vi "stage_control_mit_speichern.vi"() -> ()   [LabVIEW 2009]
uses:
  global_stage_initialised.vi
  <vilib>/Utility/inputDevices.llb/joystickAcquire.vi
  <vilib>/Utility/inputDevices.llb/closeJoystick.vi
panel:
  in  "Löschen":bool
  in  "Zeile":dbl
  out "Favoriten":i32[](listbox)
  in  "Laden":bool
  in  "Beschreibung":string
  in  "Speichern":bool
  in  "Wellenlänge":string
  in  "Joystick Index":i32
  in  "SN von Controller 1":string="0135500571"
  in  "Position auslesen":bool
  out "Joystickauslese":T1(ring)
  out "X-Achse pos/neg fahren":i32 min=-3000 max=2000
  out "Y-Achse pos/neg fahren":i32 min=-3000 max=2000
  in  "Schrittweite verringern":bool
  in  "Schrittweite erhoehen":bool
  out "Z-Achse pos fahren":bool
  out "Z-Achse neg fahren":bool
  out "Joystick ID":refnum<k1> caption="Geräte-ID"
  out "z-Achse":i32
  out "y-Achse":i32
  out "x-Achse":i32
  in  "Schrittweite [µm]":u16(ring) items=["500,0", "200,0", "100,0", "50,0", "20,0", "10,0", "5,0", "2,0", "1,0", "0,5", "0,1"]
  out "Aktuelle xyz-Position [mm]":dbl[](array[numeric]) format="%.5g"
  in  "Geschwindigkeit einstellen":bool
  in  "Ziel Geschwindigkeit [mm/s]":dbl=0.3 min=0.01 max=0.6 step=0.001 format="%.3g"
  out "Geschwindigkeit [mm/s]":dbl format="%.3g"
  in  "Negativer Schritt":bool[](array[boolean])
  in  "Positiver Schritt":bool[](array[boolean])
  out "error out":errorcluster
  out "Achse in \nBewegung":bool
  in  "Ziel xyz-Position [mm]":dbl[](array[numeric]) step=1e-05 format="%.5g"
  out "xyz-Bezeichnung":string[](array[string])=["x [mm]", "y [mm]", "z [mm]"]
  in  "Bühnen schließen":bool
  out "Bühnen\ninitialisiert":bool
  # "Steuerung der 3D-Translationsbühne von PI"
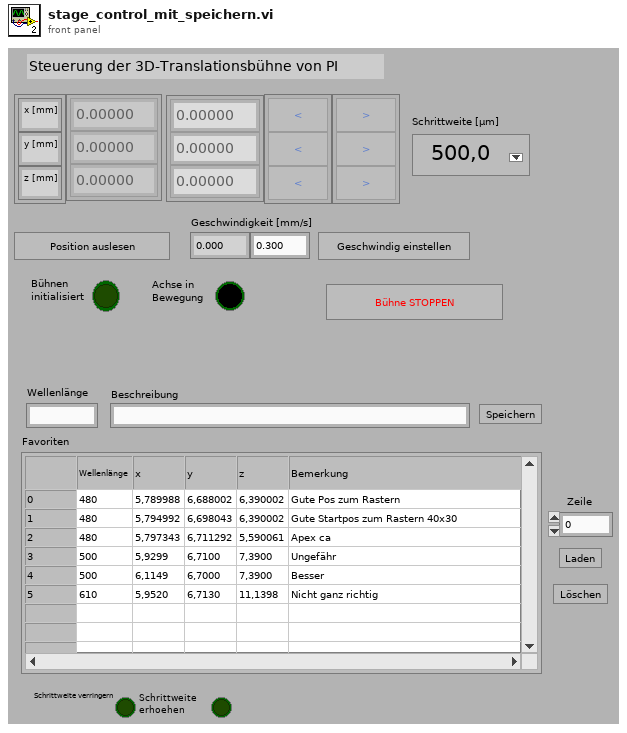
[diagram p1: front panel]
types:
  T1 = enum16{"Nichts tun", "X-Achse", "Y-Achse", "Z-Achse positiv", "Z-Achse negativ", "Schrittweite erhoehen", "Schrittweite verringern"}
  T2 = cluster{"Objektnamen":string[][], "Zeilentitel":string[], "Spaltentitel":string[]}
  T3 = cluster{"X axis":i32, "Y axis":i32, "Z axis":i32, "X axis rotation":i32, "Y axis rotation":i32, "Z axis rotation":i32, "U axis":i32, "V axis":i32}
  T4 = cluster{"button 1":bool, "button 2":bool, "button 3":bool, "button 4":bool, "button 5":bool, "button 6":bool, "button 7":bool, "button 8":bool, "button 9":bool, "button 10":bool, "button 11":bool, "button 12":bool, "button 13":bool, "button 14":bool, "button 15":bool, "button 16":bool, "button 17":bool, "button 18":bool, "button 19":bool, "button 20":bool, "button 21":bool, "button 22":bool, "button 23":bool, "button 24":bool, "button 25":bool, "button 26":bool, "button 27":bool, "button 28":bool, "button 29":bool, "button 30":bool, "button 31":bool, "button 32":bool}
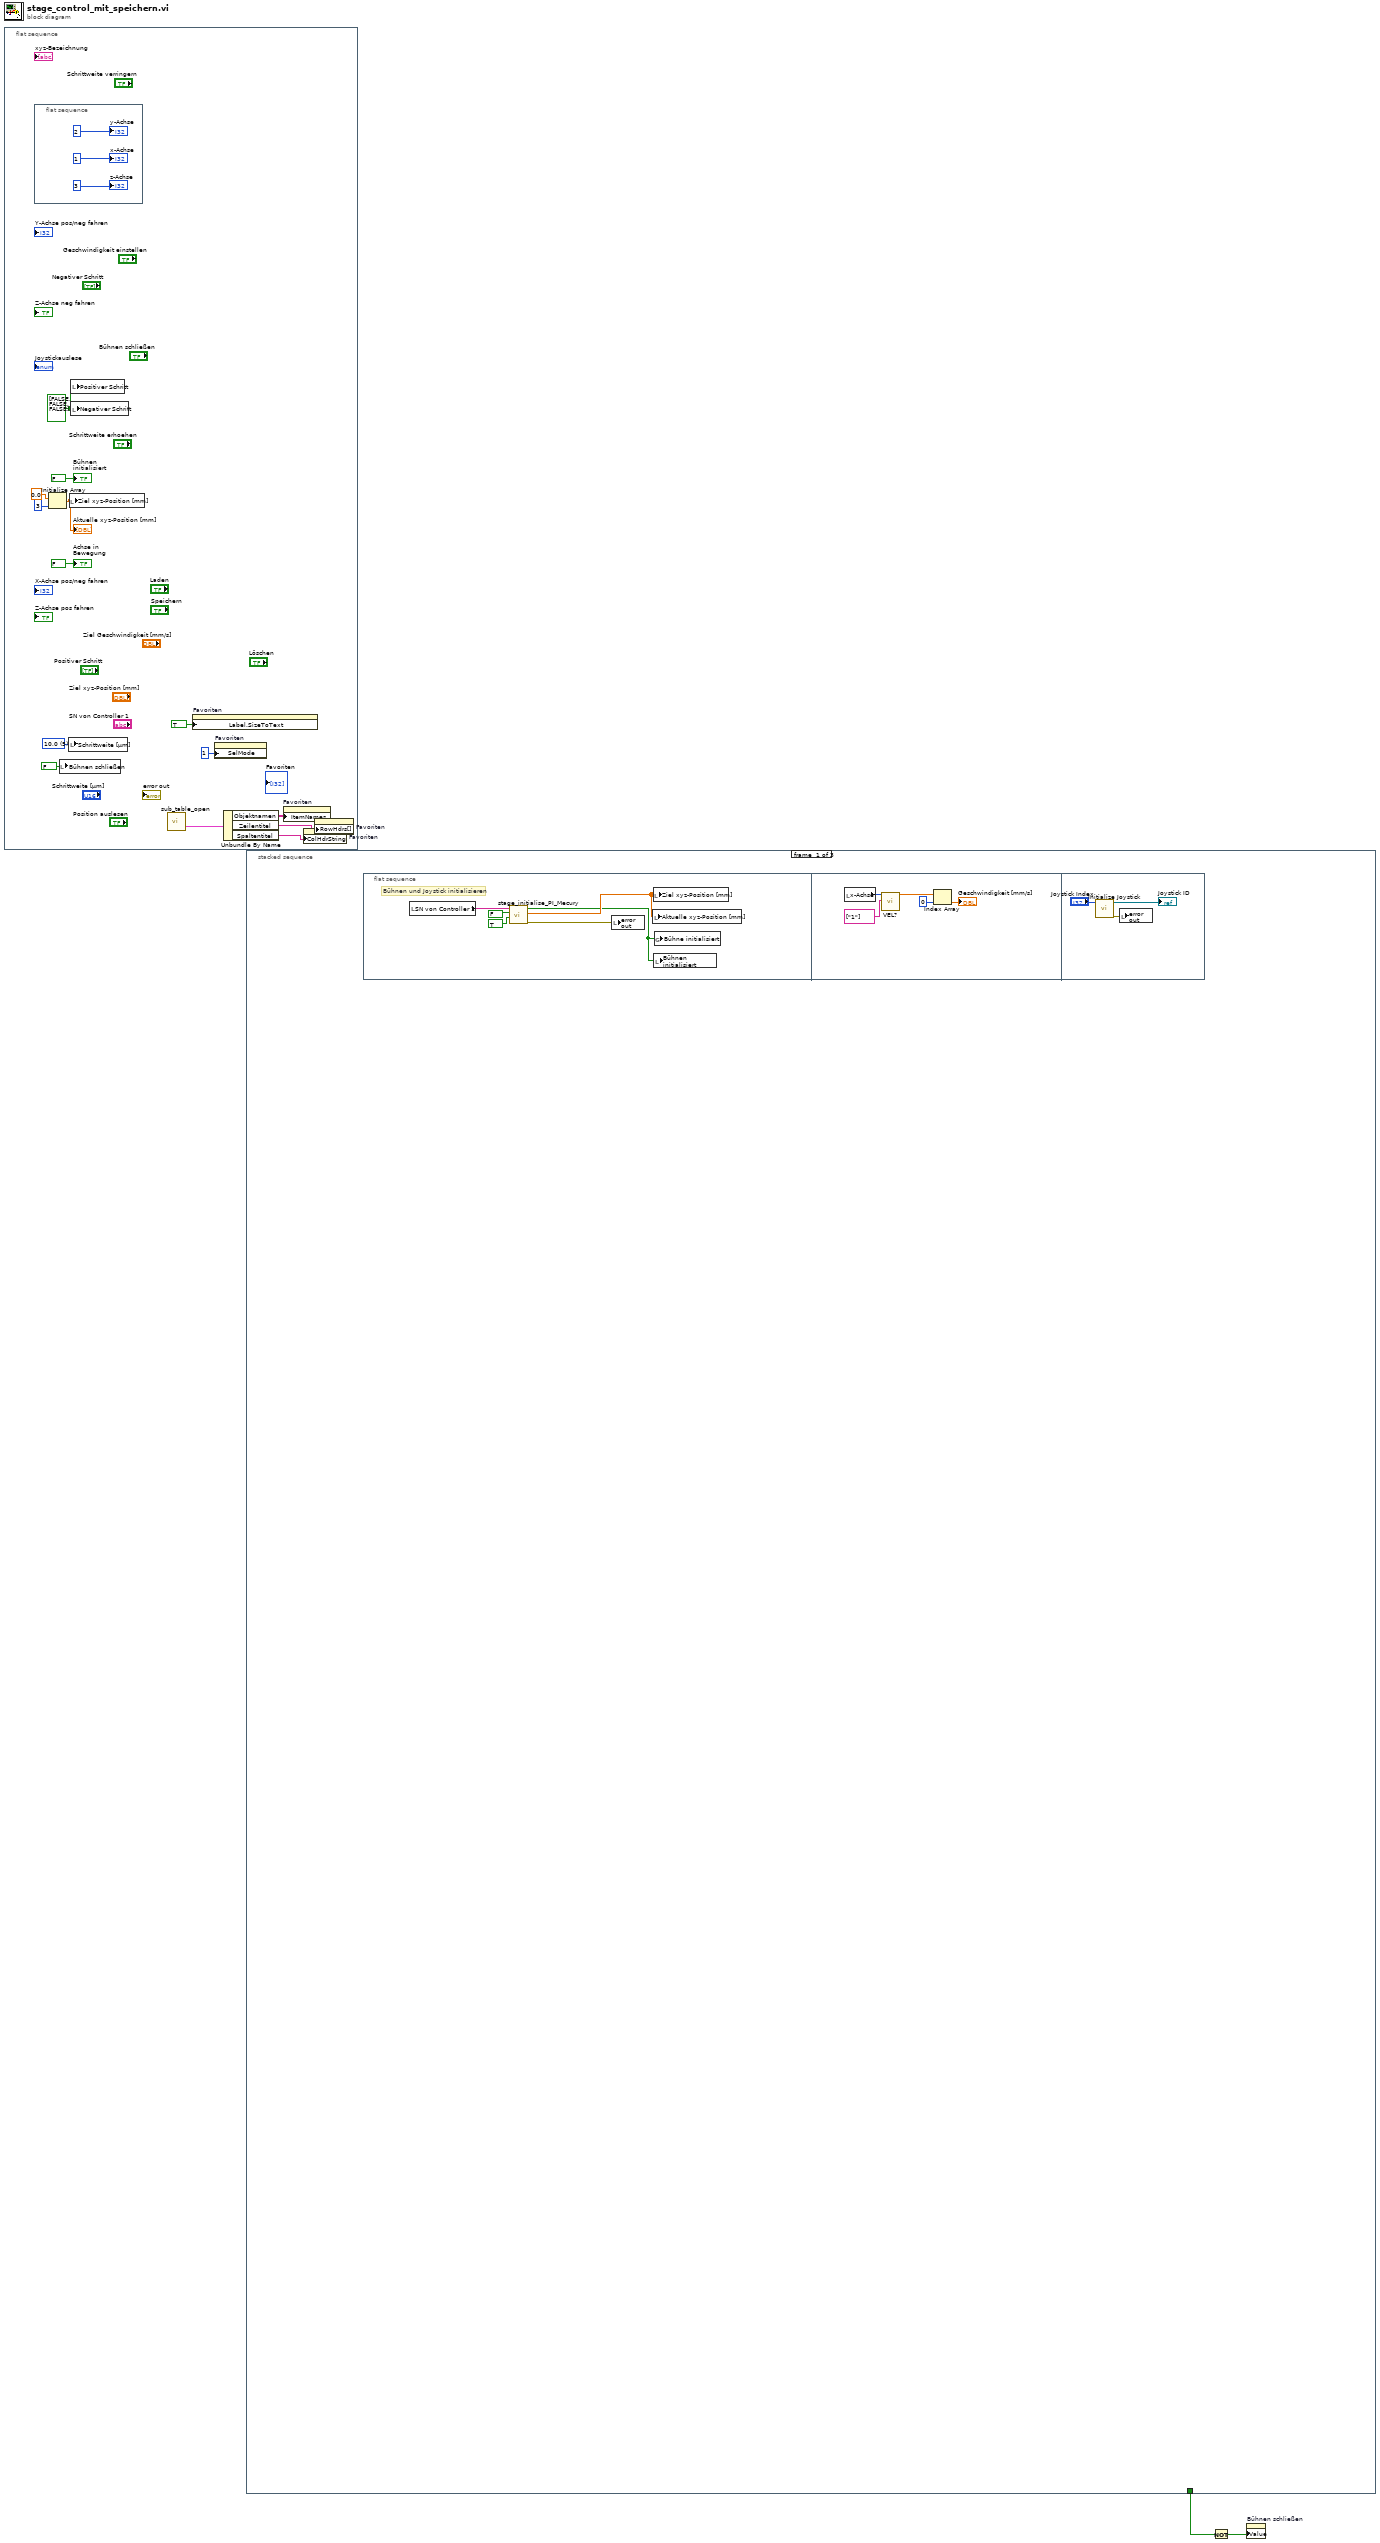
[diagram p0: block diagram]
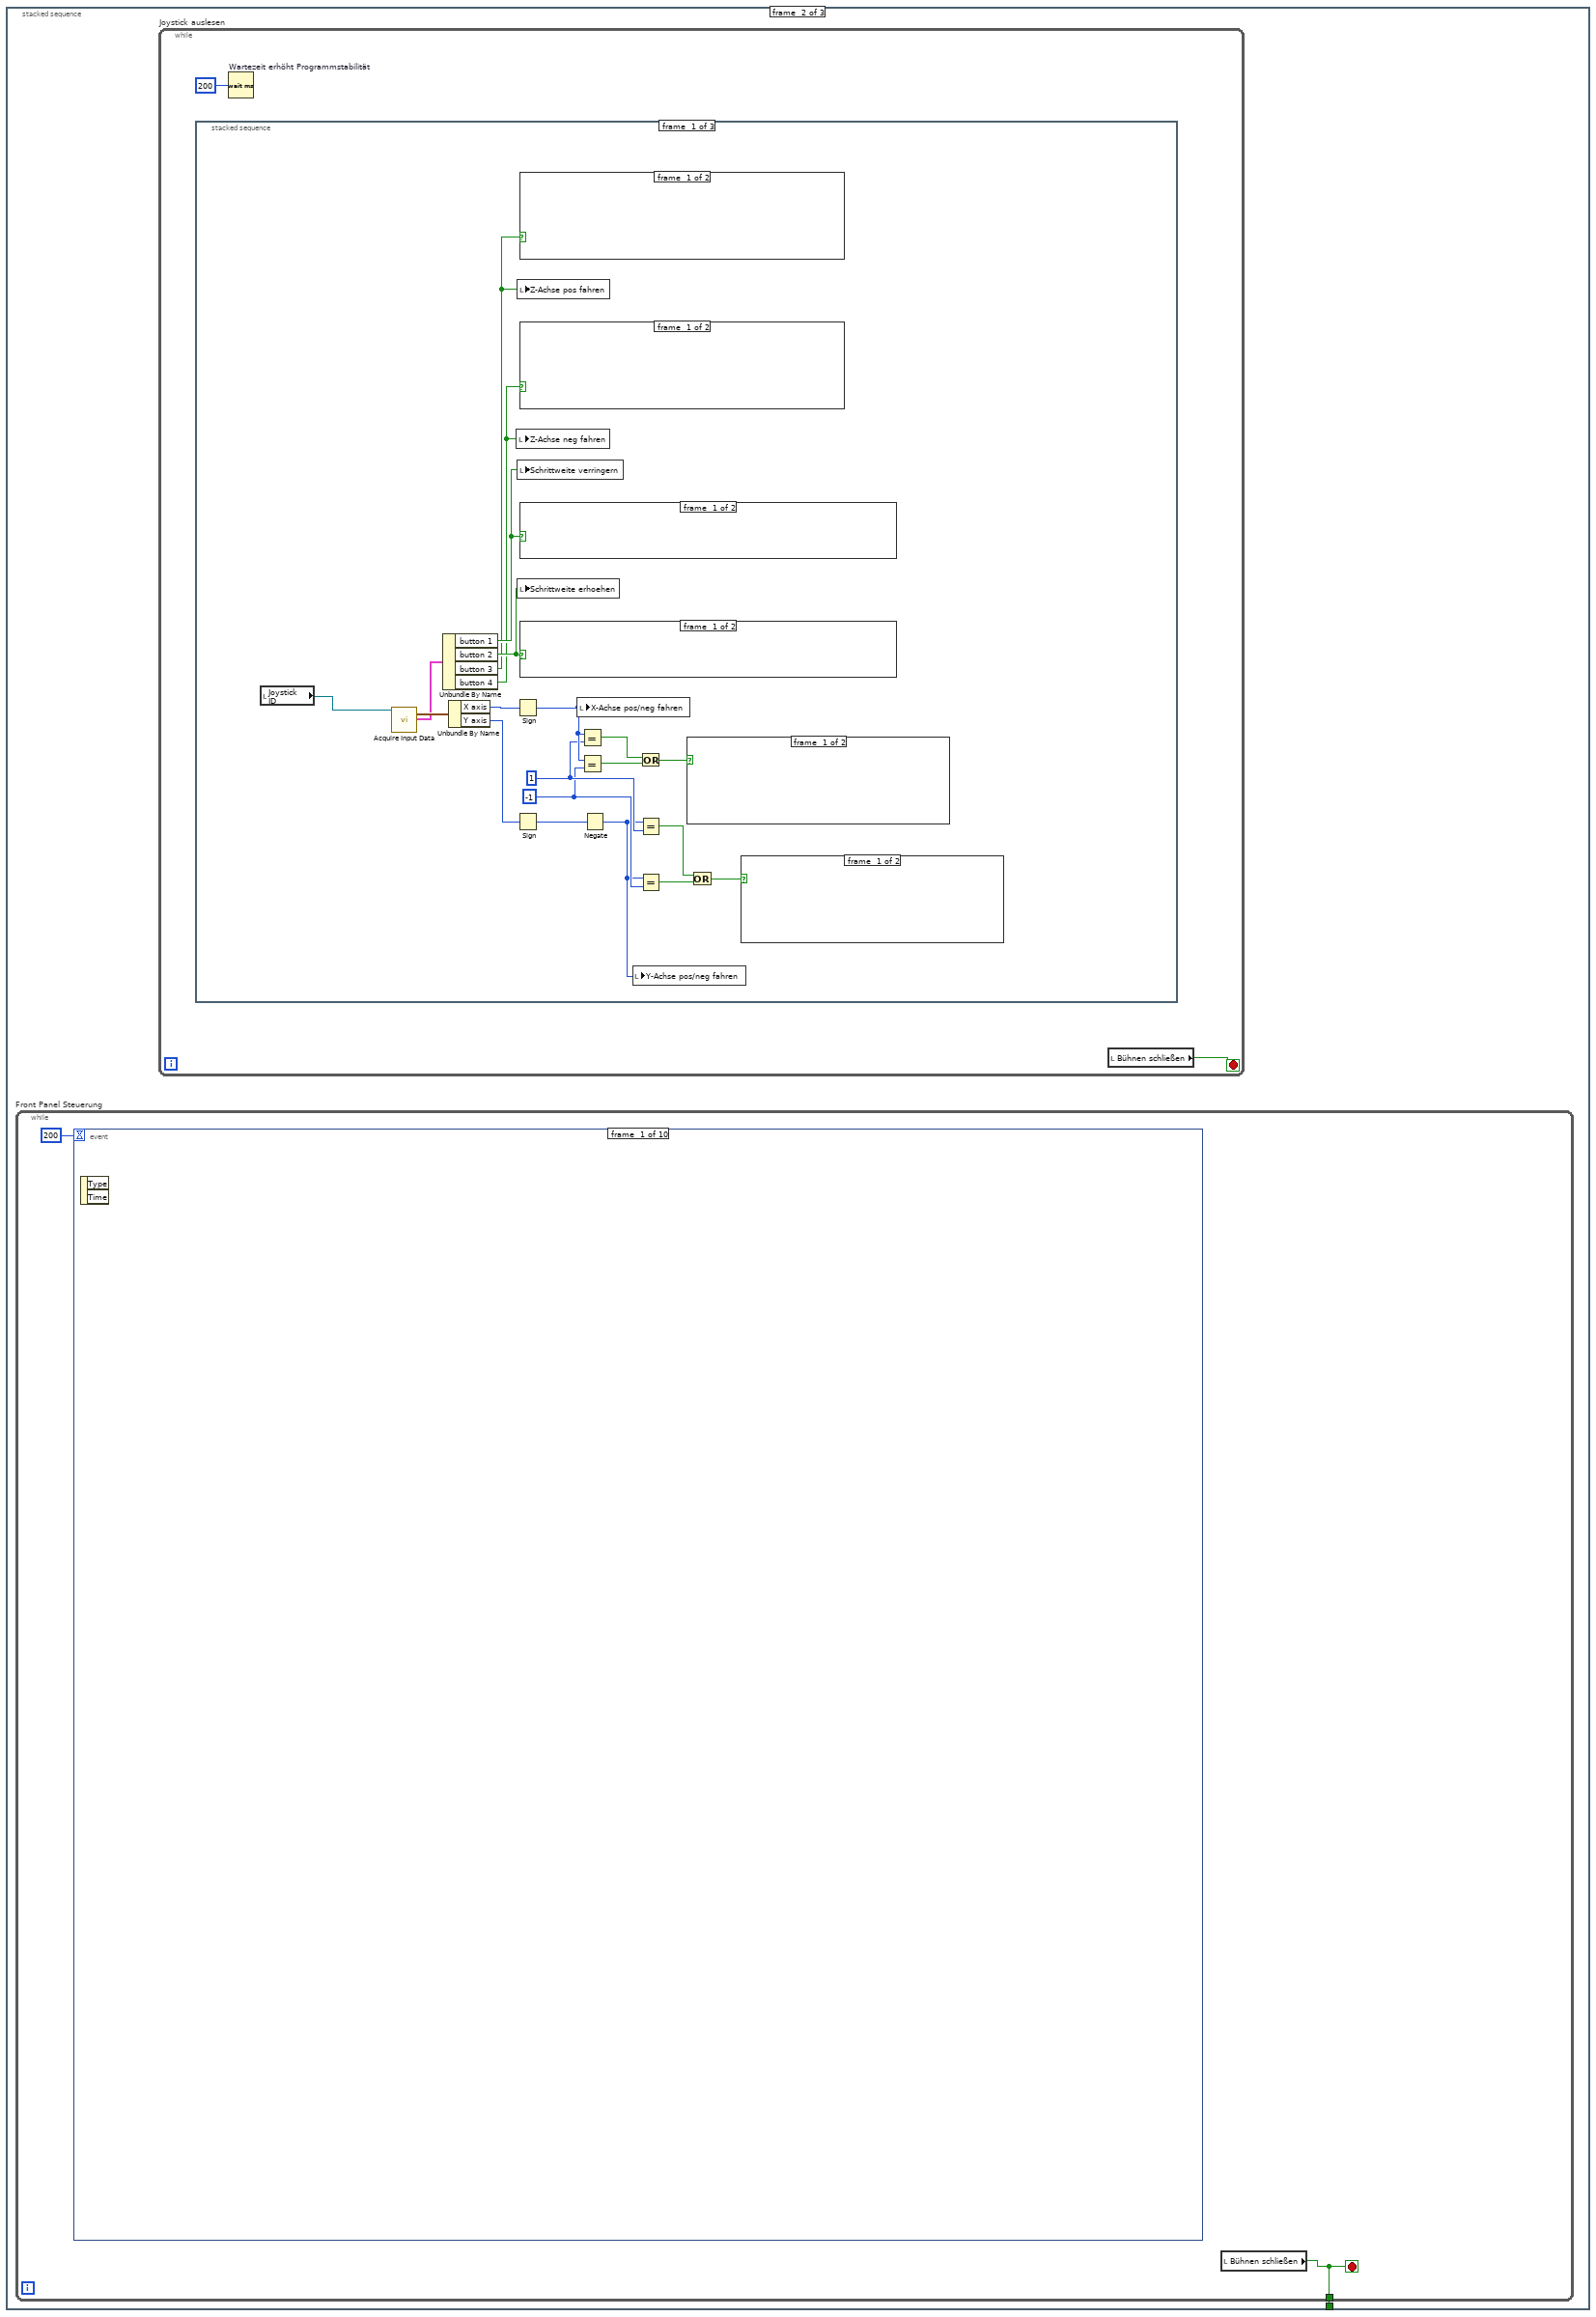
[diagram p2: hidden frame]
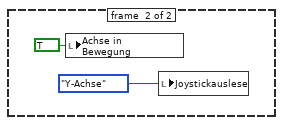
[diagram p3: hidden frame]
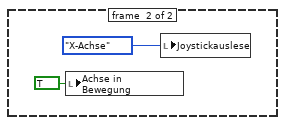
[diagram p4: hidden frame]
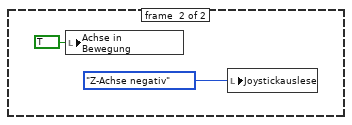
[diagram p5: hidden frame]
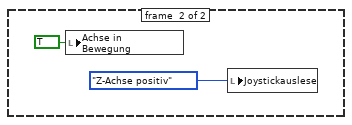
[diagram p6: hidden frame]
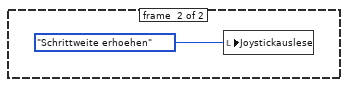
[diagram p7: hidden frame]
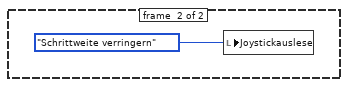
[diagram p8: hidden frame]
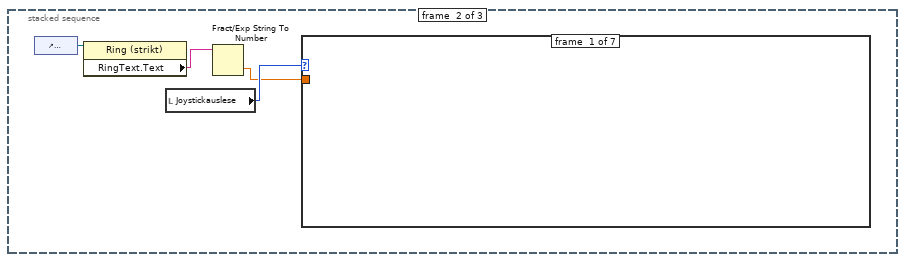
[diagram p9: hidden frame]
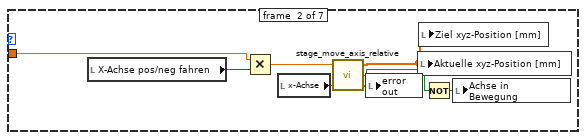
[diagram p10: hidden frame]
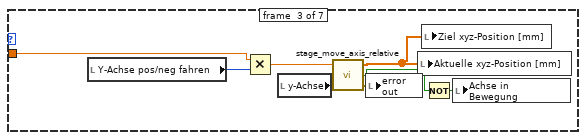
[diagram p11: hidden frame]
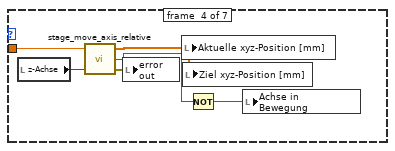
[diagram p12: hidden frame]
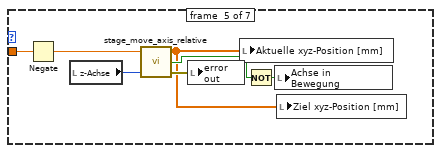
[diagram p13: hidden frame]
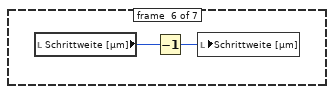
[diagram p14: hidden frame]
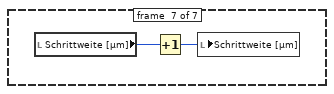
[diagram p15: hidden frame]
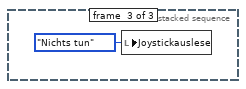
[diagram p16: hidden frame]
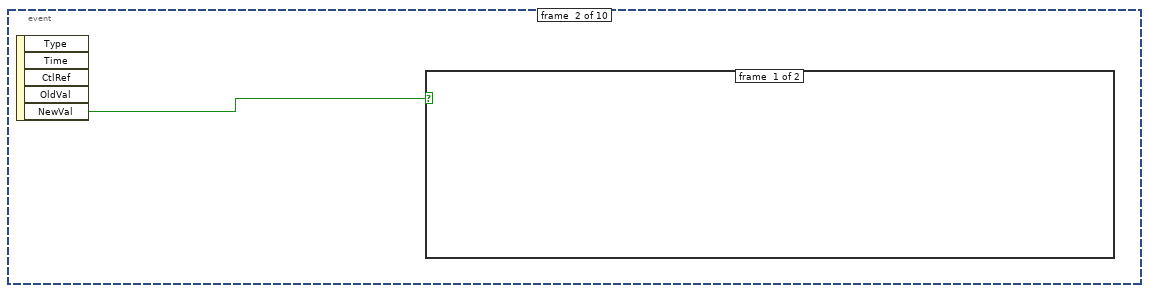
[diagram p17: hidden frame]
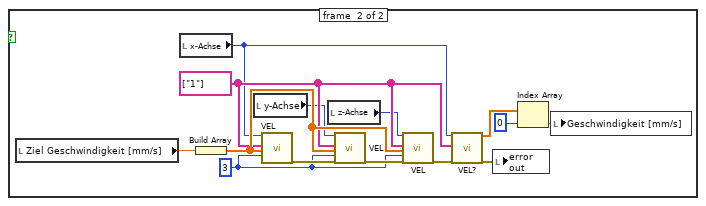
[diagram p18: hidden frame]
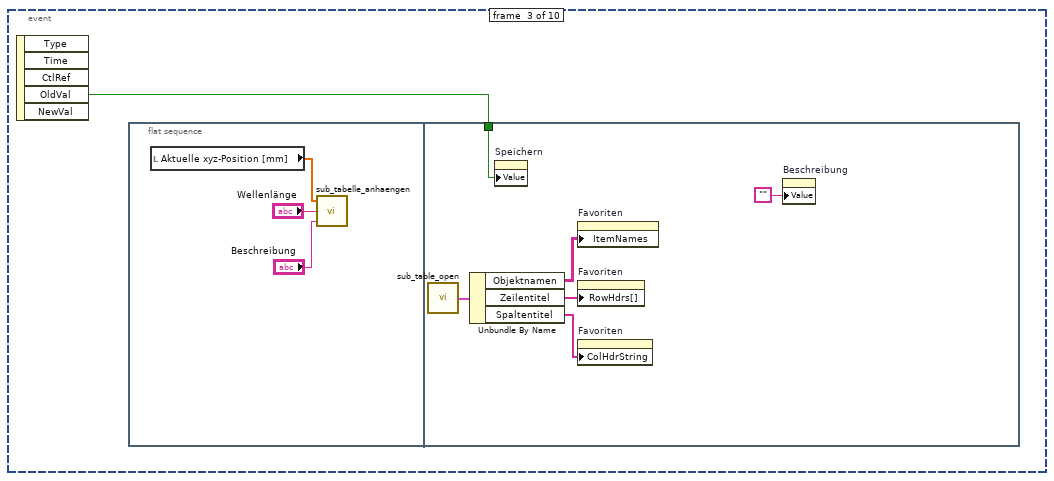
[diagram p19: hidden frame]
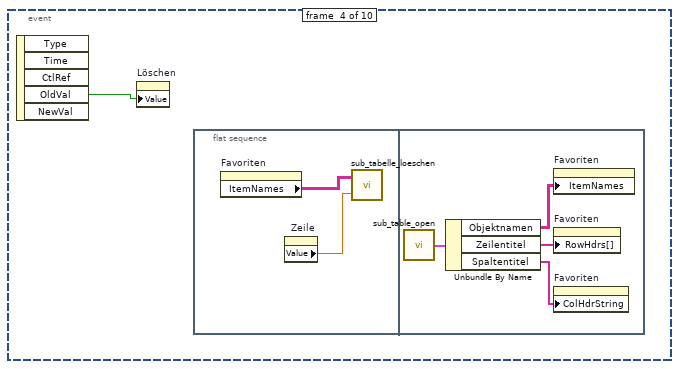
[diagram p20: hidden frame]
diagram:
  n1 = flat-sequence {
    frame #0 {
      w15 = u16 5 items=["500,0", "200,0", "100,0", "50,0", "20,0", "10,0", "5,0", "2,0", "1,0", "0,5"] ("Schrittweite [µm]")
      w11 = bool[] [FALSE, FALSE, FALSE] ("Positiver Schritt")
      n2 = flat-sequence {
        frame #0 {
          "x-Achse" <- 1 ("x-Achse")
          "y-Achse" <- 2 ("y-Achse")
          "z-Achse" <- 3 ("z-Achse")
        }
      }
      n3 = Initialize Array(0.0 ("Element"), 3 ("Dimension")) -> (w14:dbl[])
      "Aktuelle xyz-Position [mm]" <- w14
      n4 = local write "Bühnen schließen"(FALSE ("Bühnen schließen")) -> ()
      n5 = local write "Schrittweite [µm]"(w15) -> ()
      n6 = local write "Ziel xyz-Position [mm]"(w14) -> ()
      n7 = local write "Positiver Schritt"(w11) -> ()
      n8 = local write "Negativer Schritt"(w11) -> ()
      n9 = call "sub_table_open.vi"() -> ("Cluster (Ausgang)"=w6:T2)  [unwired: 1 in]
      n10 = property on="Favoriten" class="MehrSpaltListenfeld (strikt)"("Label.SizeToText"=TRUE ("Beschriftung.Größe an Text anpassen?")) -> ()  [unwired: 2 in, 2 out]
      n11 = property on="Favoriten" class="MehrSpaltListenfeld (strikt)"("SelMode"=1 ("Auswahlmodus")) -> ()  [unwired: 2 in, 2 out]
      n12 = Unbundle By Name(w6) -> ("Objektnamen"=w5:string[][], "Zeilentitel"=w3:string[], "Spaltentitel"=w4:string[])
      n13 = property on="Favoriten" class="MehrSpaltListenfeld (strikt)"("ItemNames"=w5) -> ()  [unwired: 2 in, 2 out]
      n14 = property on="Favoriten" class="MehrSpaltListenfeld (strikt)"("ColHdrString"=w4) -> ()  [unwired: 2 in, 2 out]
      n15 = property on="Favoriten" class="MehrSpaltListenfeld (strikt)"("RowHdrs[]"=w3) -> ()  [unwired: 2 in, 2 out]
      "Bühnen\ninitialisiert" <- FALSE ("Bühnen initialisiert")
      "Achse in \nBewegung" <- FALSE ("x-Achse in Bewegung")
    }
  }
  n16 = stacked-sequence {
    tunnel: [_ w34 _] -> w2
    frame #0 {
      n17 = flat-sequence {
        frame #0 {
          # "Bühnen und Joystick initialisieren"
          n18 = local read "SN von Controller 1"() -> (w20:string)
          n19 = call "stage_initialise_PI_Mecury.vi"("Referenz Modus"=TRUE, "Referenzierung erzwingen"=FALSE, "SN von Controller 1"=w20) -> ("error out"=w23:errorcluster, "Aktuelle xyz-Position"=w22:dbl[], "Bühnen initialisiert"=w21:bool)  [unwired: 6 in]
          n20 = local write "error out"(w23) -> ()
          n21 = local write "Aktuelle xyz-Position [mm]"(w22) -> ()
          n22 = local write "Ziel xyz-Position [mm]"(w22) -> ()
          n23 = local write "Bühnen\ninitialisiert"(w21) -> ()
          n24 = global write "global_stage_initialised.vi" "Bühne initialisiert"(w21) -> ()
        }
        frame #1 {
          n25 = local read "x-Achse"() -> (w26:i32)
          n26 = call "VEL?.vi"("System no."=w26, "Axes to query"=string[] ["1"]) -> ("Velocity"=w27:dbl[])  [unwired: 16 in, 1 out]
          n27 = Index Array(array=w27, index=0 ("Index")) -> (element=→"Geschwindigkeit [mm/s]":dbl)
        }
        frame #2 {
          n28 = call <vilib>:"Initialize Joystick.vi"("device index"="Joystick Index") -> ("error out"=w32:errorcluster, "device ID"=→"Joystick ID":refnum<k1>)  [unwired: 9 in]
          n29 = local write "error out"(w32) -> ()
        }
      }
    }
    frame #1 {
      n30 = while "Front Panel Steuerung" {
        tunnel: [w105] -> w34
        stop <- w105 stop-if-true
        n31 = event shown="[2] \"Speichern\": Wertänderung" {
          selector: _ -> [_ _ _ _ _ _ _ _ _ _]
          dyn-events: _ -> [_ _ _ _ _ _ _ _ _ _]
          timeout: 200 -> [_ _ _ _ _ _ _ _ _ _]
          event #0 {
            n32 = event-data() -> ()  [unwired: 1 in, 2 out]
          }
          event #1 {
            n33 = event-data() -> ("NewVal"=w107:bool)  [unwired: 1 in, 4 out]
            n34 = case shown="True" w107 {
              frame #0 {
              }
              frame #1 {
                w118 = i16 3 ("No.of digits")
                w114 = string[] ["1"] ("Axes to set")
                n35 = local read "Ziel Geschwindigkeit [mm/s]"() -> (w119:dbl)
                n36 = local read "x-Achse"() -> (w110:i32)
                n37 = Build Array(w119) -> (w117:dbl[])
                n38 = local read "y-Achse"() -> (w109:i32)
                n39 = call "VEL.vi"("System no."=w110, "Axes to set"=w114, "Velocity values"=w117, "No.of digits"=w118) -> ("error out"=w121:errorcluster)  [unwired: 14 in, 1 out]
                n40 = local read "z-Achse"() -> (w108:i32)
                n41 = call "VEL.vi"("System no."=w109, "Axes to set"=w114, "Velocity values"=w117, "No.of digits"=w118, "error in"=w121) -> ("error out"=w120:errorcluster)  [unwired: 13 in, 1 out]
                n42 = call "VEL.vi"("System no."=w108, "Axes to set"=w114, "Velocity values"=w117, "No.of digits"=w118, "error in"=w120) -> ("error out"=w115:errorcluster)  [unwired: 13 in, 1 out]
                n43 = call "VEL?.vi"("System no."=w110, "Axes to query"=w114, "error in"=w115) -> ("Velocity"=w112:dbl[], "error out"=w116:errorcluster)  [unwired: 15 in]
                n44 = local write "error out"(w116) -> ()
                n45 = Index Array(array=w112, index=0 ("Index")) -> (element=w113:dbl)
                n46 = local write "Geschwindigkeit [mm/s]"(w113) -> ()
              }
            }
          }
          event #2 {
            n47 = event-data() -> ("OldVal"=w122:bool)  [unwired: 1 in, 4 out]
            n48 = flat-sequence {
              tunnel: w122 -> [w130]
              frame #0 {
                n49 = local read "Aktuelle xyz-Position [mm]"() -> (w123:dbl[])
                n50 = call "sub_tabelle_anhaengen.vi"("Beschreibung"="Beschreibung", "Wellenlänge"="Wellenlänge", "Aktuelle xyz-Position [mm]"=w123) -> ()
              }
              frame #1 {
                n51 = call "sub_table_open.vi"() -> ("Cluster (Ausgang)"=w129:T2)  [unwired: 1 in]
                n52 = Unbundle By Name(w129) -> ("Objektnamen"=w128:string[][], "Zeilentitel"=w127:string[], "Spaltentitel"=w126:string[])
                n53 = property on="Speichern" class="Boolesch (strikt)"("Value"=w130) -> ()  [unwired: 2 in, 2 out]
                n54 = property on="Favoriten" class="MehrSpaltListenfeld (strikt)"("ItemNames"=w128) -> ()  [unwired: 2 in, 2 out]
                n55 = property on="Favoriten" class="MehrSpaltListenfeld (strikt)"("RowHdrs[]"=w127) -> ()  [unwired: 2 in, 2 out]
                n56 = property on="Favoriten" class="MehrSpaltListenfeld (strikt)"("ColHdrString"=w126) -> ()  [unwired: 2 in, 2 out]
                n57 = property on="Beschreibung" class="Str"("Value"="") -> ()  [unwired: 2 in, 2 out]
              }
            }
          }
          event #3 {
            n58 = event-data() -> ("OldVal"=w132:bool)  [unwired: 1 in, 4 out]
            n59 = property on="Löschen" class="Boolesch (strikt)"("Value"=w132) -> ()  [unwired: 2 in, 2 out]
            n60 = flat-sequence {
              frame #0 {
                n61 = property on="Favoriten" class="MehrSpaltListenfeld (strikt)"() -> ("ItemNames"=w133:string[][])  [unwired: 2 in, 2 out]
                n62 = property on="Zeile" class="DigitalWert (strikt)"() -> ("Value"=w134:dbl)  [unwired: 2 in, 2 out]
                n63 = call "sub_tabelle_loeschen.vi"("Numerisches Element"=w134, "Array"=w133) -> ()  [unwired: 1 in]
              }
              frame #1 {
                n64 = call "sub_table_open.vi"() -> ("Cluster (Ausgang)"=w138:T2)  [unwired: 1 in]
                n65 = Unbundle By Name(w138) -> ("Objektnamen"=w135:string[][], "Zeilentitel"=w137:string[], "Spaltentitel"=w136:string[])
                n66 = property on="Favoriten" class="MehrSpaltListenfeld (strikt)"("ItemNames"=w135) -> ()  [unwired: 2 in, 2 out]
                n67 = property on="Favoriten" class="MehrSpaltListenfeld (strikt)"("RowHdrs[]"=w137) -> ()  [unwired: 2 in, 2 out]
                n68 = property on="Favoriten" class="MehrSpaltListenfeld (strikt)"("ColHdrString"=w136) -> ()  [unwired: 2 in, 2 out]
              }
            }
          }
          event #4 {
            n69 = event-data() -> ("OldVal"=w141:bool)  [unwired: 1 in, 4 out]
            n70 = local write "Laden"(w141) -> ()
            n71 = property on="Favoriten" class="MehrSpaltListenfeld (strikt)"() -> ("ItemNames"=w140:string[][])  [unwired: 2 in, 2 out]
            n72 = call "sub_table_laden.vi"("Zeile"="Zeile", "ItemNames"=w140) -> ("Array"=w139:dbl[])
            n73 = property on="Ziel xyz-Position [mm]" class="Arr (strikt)"("Val(Sgnl)"=w139) -> ()  [unwired: 2 in, 2 out]
          }
          event #5 {
            n74 = event-data() -> ("NewVal"=w143:bool)  [unwired: 1 in, 4 out]
            n75 = case shown="True" w143 {
              frame #0 {
              }
              frame #1 {
                n76 = call "stage_get_current_xyz.vi"() -> ("error out"=w145:errorcluster, "Aktuelle xyz-Position OUT [mm]"=w144:dbl[])  [unwired: 3 in]
                n77 = local write "Aktuelle xyz-Position [mm]"(w144) -> ()
                n78 = local write "error out"(w145) -> ()
                n79 = local write "Ziel xyz-Position [mm]"(w144) -> ()
              }
            }
          }
          event #6 {
            n80 = event-data() -> ("OldVal"=w147:dbl[], "NewVal"=w146:dbl[])  [unwired: 1 in, 3 out]
            n81 = flat-sequence {
              tunnel: [w153] -> w150
              tunnel: [w152] -> w149
              tunnel: [w151] -> w148
              tunnel: w147 -> [w155]
              tunnel: w146 -> [w154]
              tunnel: w150 -> [w169]
              tunnel: w149 -> [w168]
              tunnel: w148 -> [w167]
              frame #0 {
                w158 = 2 ("Index")
                w157 = 1 ("Index")
                w156 = 0 ("Index")
                # "Änderung des Ziels: Entscheide welche Achse gefahren werden soll"
                n82 = local write "Achse in \nBewegung"(TRUE ("x-Achse in Bewegung")) -> ()
                n83 = Index Array(array=w155, index #1=w156, index #2=w157, index #3=w158) -> (element #1=w159:dbl, element #2=w160:dbl, element #3=w163:dbl)
                n84 = Index Array(array=w154, index #1=w156, index #2=w157, index #3=w158) -> (element #1=w164:dbl, element #2=w161:dbl, element #3=w162:dbl)
                n85 = Not Equal?(x=w159, y=w164) -> (x != y?=w153:bool)
                n86 = Not Equal?(x=w160, y=w161) -> (x != y?=w152:bool)
                n87 = Not Equal?(x=w163, y=w162) -> (x != y?=w151:bool)
              }
              frame #1 {
                n88 = local read "Ziel xyz-Position [mm]"() -> (w166:dbl[])
                n89 = case shown="True" w169 {
                  tunnel: w166 -> [_ w186]
                  frame #0 {
                  }
                  frame #1 {
                    n90 = local read "x-Achse"() -> (w184:i32)
                    n91 = call "stage_move_axis_absolute.vi"("Ziel xyz IN [mm]"=w186, "Achse"=w184) -> ("error out"=w187:errorcluster, "Fertig?"=w185:bool, "Ziel xyz OUT [mm]"=w182:dbl[])  [unwired: 1 in]
                    n92 = local write "Aktuelle xyz-Position [mm]"(w182) -> ()
                    n93 = local write "Ziel xyz-Position [mm]"(w182) -> ()
                    n94 = local write "error out"(w187) -> ()
                    n95 = Not(x=w185) -> (.not. x?=w183:bool)
                    n96 = local write "Achse in \nBewegung"(w183) -> ()
                  }
                }
                n97 = case shown="True" w168 {
                  tunnel: w166 -> [_ w180]
                  frame #0 {
                  }
                  frame #1 {
                    n98 = local read "y-Achse"() -> (w178:i32)
                    n99 = call "stage_move_axis_absolute.vi"("Ziel xyz IN [mm]"=w180, "Achse"=w178) -> ("error out"=w181:errorcluster, "Fertig?"=w179:bool, "Ziel xyz OUT [mm]"=w176:dbl[])  [unwired: 1 in]
                    n100 = local write "Aktuelle xyz-Position [mm]"(w176) -> ()
                    n101 = local write "Ziel xyz-Position [mm]"(w176) -> ()
                    n102 = local write "error out"(w181) -> ()
                    n103 = Not(x=w179) -> (.not. x?=w177:bool)
                    n104 = local write "Achse in \nBewegung"(w177) -> ()
                  }
                }
                n105 = case shown="True" w167 {
                  tunnel: w166 -> [_ w173]
                  frame #0 {
                  }
                  frame #1 {
                    n106 = local read "z-Achse"() -> (w172:i32)
                    n107 = call "stage_move_axis_absolute.vi"("Ziel xyz IN [mm]"=w173, "Achse"=w172) -> ("error out"=w175:errorcluster, "Fertig?"=w174:bool, "Ziel xyz OUT [mm]"=w170:dbl[])  [unwired: 1 in]
                    n108 = local write "Aktuelle xyz-Position [mm]"(w170) -> ()
                    n109 = local write "Ziel xyz-Position [mm]"(w170) -> ()
                    n110 = local write "error out"(w175) -> ()
                    n111 = Not(x=w174) -> (.not. x?=w171:bool)
                    n112 = local write "Achse in \nBewegung"(w171) -> ()
                  }
                }
              }
            }
          }
          event #7 {
            n113 = event-data() -> ("Row"=w188:i32)  [unwired: 1 in, 7 out]
            n114 = local write "Zeile"(w188) -> ()
          }
          event #8 {
            n115 = event-data() -> ("NewVal"=w193:bool[])  [unwired: 1 in, 4 out]
            n116 = Index Array(array=w193, index #1=0 ("Index"), index #2=1 ("Index"), index #3=2 ("Index")) -> (element #1=w191:bool, element #2=w190:bool, element #3=w189:bool)
            n117 = Compound Arithmetic op=OR(w191, w190, w189) -> (w192:bool)
            n118 = case shown="True" w192 {
              tunnel: w191 -> [_ w199]
              tunnel: w190 -> [_ w198]
              tunnel: w189 -> [_ w197]
              frame #0 {
              }
              frame #1 {
                n119 = flat-sequence {
                  tunnel: [w202] -> w200
                  tunnel: w200 -> [w208]
                  tunnel: w199 -> [w207]
                  tunnel: w198 -> [w206]
                  tunnel: w197 -> [w205]
                  frame #0 {
                    n120 = local write "Achse in \nBewegung"(TRUE ("Achse in Bewegung")) -> ()
                    n121 = control-ref of="Schrittweite [µm]"() -> (w204:refnum<vi>)
                    n122 = property class="Ring (strikt)"(reference=w204) -> ("RingText.Text"=w203:string)  [unwired: 1 in, 2 out]
                    n123 = Fract/Exp String To Number(string=w203) -> (number=w202:dbl)  [unwired: 3 in, 1 out]
                  }
                  frame #1 {
                    n124 = local read "x-Achse"() -> (w211:i32)
                    n125 = local read "y-Achse"() -> (w209:i32)
                    n126 = local read "z-Achse"() -> (w210:i32)
                    n127 = case shown="True" w205 {
                      tunnel: w210 -> [_ w217]
                      tunnel: w208 -> [_ w213]
                      frame #0 {
                      }
                      frame #1 {
                        n128 = call "stage_move_axis_relative.vi"("Achse"=w217, "Schrittweite [µm]"=w213) -> ("error out"=w216:errorcluster, "Fertig?"=w215:bool, "xyz-Position OUT [mm]"=w212:dbl[])  [unwired: 1 in]
                        n129 = local write "Aktuelle xyz-Position [mm]"(w212) -> ()
                        n130 = local write "Ziel xyz-Position [mm]"(w212) -> ()
                        n131 = local write "error out"(w216) -> ()
                        n132 = Not(x=w215) -> (.not. x?=w214:bool)
                        n133 = local write "Achse in \nBewegung"(w214) -> ()
                      }
                    }
                    n134 = case shown="True" w206 {
                      tunnel: w209 -> [_ w222]
                      tunnel: w208 -> [_ w219]
                      frame #0 {
                      }
                      frame #1 {
                        n135 = call "stage_move_axis_relative.vi"("Achse"=w222, "Schrittweite [µm]"=w219) -> ("error out"=w223:errorcluster, "Fertig?"=w221:bool, "xyz-Position OUT [mm]"=w218:dbl[])  [unwired: 1 in]
                        n136 = local write "Aktuelle xyz-Position [mm]"(w218) -> ()
                        n137 = local write "Ziel xyz-Position [mm]"(w218) -> ()
                        n138 = local write "error out"(w223) -> ()
                        n139 = Not(x=w221) -> (.not. x?=w220:bool)
                        n140 = local write "Achse in \nBewegung"(w220) -> ()
                      }
                    }
                    n141 = case shown="True" w207 {
                      tunnel: w211 -> [_ w228]
                      tunnel: w208 -> [_ w225]
                      frame #0 {
                      }
                      frame #1 {
                        n142 = call "stage_move_axis_relative.vi"("Achse"=w228, "Schrittweite [µm]"=w225) -> ("error out"=w229:errorcluster, "Fertig?"=w227:bool, "xyz-Position OUT [mm]"=w224:dbl[])  [unwired: 1 in]
                        n143 = local write "Aktuelle xyz-Position [mm]"(w224) -> ()
                        n144 = local write "Ziel xyz-Position [mm]"(w224) -> ()
                        n145 = local write "error out"(w229) -> ()
                        n146 = Not(x=w227) -> (.not. x?=w226:bool)
                        n147 = local write "Achse in \nBewegung"(w226) -> ()
                      }
                    }
                  }
                }
              }
            }
          }
          event #9 {
            n148 = event-data() -> ("NewVal"=w234:bool[])  [unwired: 1 in, 4 out]
            n149 = Index Array(array=w234, index #1=0 ("Index"), index #2=1 ("Index"), index #3=2 ("Index")) -> (element #1=w232:bool, element #2=w231:bool, element #3=w230:bool)
            n150 = Compound Arithmetic op=OR(w232, w231, w230) -> (w233:bool)
            n151 = case shown="True" w233 {
              tunnel: w232 -> [_ w240]
              tunnel: w231 -> [_ w239]
              tunnel: w230 -> [_ w238]
              frame #0 {
              }
              frame #1 {
                n152 = flat-sequence {
                  tunnel: [w244] -> w241
                  tunnel: w241 -> [w250]
                  tunnel: w240 -> [w249]
                  tunnel: w239 -> [w248]
                  tunnel: w238 -> [w247]
                  frame #0 {
                    n153 = local write "Achse in \nBewegung"(TRUE ("Achse in Bewegung")) -> ()
                    n154 = control-ref of="Schrittweite [µm]"() -> (w246:refnum<vi>)
                    n155 = property class="Ring (strikt)"(reference=w246) -> ("RingText.Text"=w245:string)  [unwired: 1 in, 2 out]
                    n156 = Fract/Exp String To Number(string=w245) -> (number=w243:dbl)  [unwired: 3 in, 1 out]
                    n157 = Negate(x=w243) -> (-x=w244:dbl)
                  }
                  frame #1 {
                    n158 = local read "x-Achse"() -> (w251:i32)
                    n159 = local read "y-Achse"() -> (w252:i32)
                    n160 = local read "z-Achse"() -> (w253:i32)
                    n161 = case shown="True" w247 {
                      tunnel: w253 -> [_ w259]
                      tunnel: w250 -> [_ w255]
                      frame #0 {
                      }
                      frame #1 {
                        n162 = call "stage_move_axis_relative.vi"("Achse"=w259, "Schrittweite [µm]"=w255) -> ("error out"=w258:errorcluster, "Fertig?"=w257:bool, "xyz-Position OUT [mm]"=w254:dbl[])  [unwired: 1 in]
                        n163 = local write "Aktuelle xyz-Position [mm]"(w254) -> ()
                        n164 = local write "Ziel xyz-Position [mm]"(w254) -> ()
                        n165 = local write "error out"(w258) -> ()
                        n166 = Not(x=w257) -> (.not. x?=w256:bool)
                        n167 = local write "Achse in \nBewegung"(w256) -> ()
                      }
                    }
                    n168 = case shown="True" w248 {
                      tunnel: w252 -> [_ w264]
                      tunnel: w250 -> [_ w261]
                      frame #0 {
                      }
                      frame #1 {
                        n169 = call "stage_move_axis_relative.vi"("Achse"=w264, "Schrittweite [µm]"=w261) -> ("error out"=w265:errorcluster, "Fertig?"=w263:bool, "xyz-Position OUT [mm]"=w260:dbl[])  [unwired: 1 in]
                        n170 = local write "Aktuelle xyz-Position [mm]"(w260) -> ()
                        n171 = local write "Ziel xyz-Position [mm]"(w260) -> ()
                        n172 = local write "error out"(w265) -> ()
                        n173 = Not(x=w263) -> (.not. x?=w262:bool)
                        n174 = local write "Achse in \nBewegung"(w262) -> ()
                      }
                    }
                    n175 = case shown="True" w249 {
                      tunnel: w251 -> [_ w270]
                      tunnel: w250 -> [_ w267]
                      frame #0 {
                      }
                      frame #1 {
                        n176 = call "stage_move_axis_relative.vi"("Achse"=w270, "Schrittweite [µm]"=w267) -> ("error out"=w271:errorcluster, "Fertig?"=w269:bool, "xyz-Position OUT [mm]"=w266:dbl[])  [unwired: 1 in]
                        n177 = local write "Aktuelle xyz-Position [mm]"(w266) -> ()
                        n178 = local write "Ziel xyz-Position [mm]"(w266) -> ()
                        n179 = local write "error out"(w271) -> ()
                        n180 = Not(x=w269) -> (.not. x?=w268:bool)
                        n181 = local write "Achse in \nBewegung"(w268) -> ()
                      }
                    }
                  }
                }
              }
            }
          }
        }
        n182 = local read "Bühnen schließen"() -> (w105:bool)
      }
      n183 = while "Joystick auslesen" {
        stop <- w36 stop-if-true
        n184 = stacked-sequence {
          frame #0 {
            w41 = -1
            w42 = 1
            n185 = local read "Joystick ID"() -> (w56:refnum<k1>)
            n186 = call-poly <vilib>:"Acquire Input Data.vi"("device ID"=w56) -> ("axis info"=w55:T3, "button info"=w54:T4)  [unwired: 14 in, 3 out]
            n187 = Unbundle By Name(w54) -> ("button 1"=w50:bool, "button 2"=w49:bool, "button 3"=w48:bool, "button 4"=w47:bool)
            n188 = Unbundle By Name(w55) -> ("X axis"=w53:i32, "Y axis"=w51:i32)
            n189 = Sign(1:w53) -> (0:w43:i32)
            n190 = Sign(1:w51) -> (0:w52:i32)
            n191 = local write "Z-Achse neg fahren"(w47) -> ()
            n192 = local write "Z-Achse pos fahren"(w48) -> ()
            n193 = local write "Schrittweite verringern"(w50) -> ()
            n194 = local write "Schrittweite erhoehen"(w49) -> ()
            n195 = case shown="True" w48 {
              frame #0 {
              }
              frame #1 {
                n196 = local write "Achse in \nBewegung"(TRUE ("Achse in Bewegung")) -> ()
                n197 = local write "Joystickauslese"(T1."Z-Achse positiv" ("Joystickauslese")) -> ()
              }
            }
            n198 = case shown="True" w47 {
              frame #0 {
              }
              frame #1 {
                n199 = local write "Achse in \nBewegung"(TRUE ("Achse in Bewegung")) -> ()
                n200 = local write "Joystickauslese"(T1."Z-Achse negativ" ("Joystickauslese")) -> ()
              }
            }
            n201 = case shown="True" w50 {
              frame #0 {
              }
              frame #1 {
                n202 = local write "Joystickauslese"(T1."Schrittweite verringern" ("Joystickauslese")) -> ()
              }
            }
            n203 = case shown="True" w49 {
              frame #0 {
              }
              frame #1 {
                n204 = local write "Joystickauslese"(T1."Schrittweite erhoehen" ("Joystickauslese")) -> ()
              }
            }
            n205 = local write "X-Achse pos/neg fahren"(w43) -> ()
            n206 = Equal?(x=w43, y=w42) -> (x = y?=w46:bool)
            n207 = Equal?(x=w43, y=w41) -> (x = y?=w45:bool)
            n208 = Negate(x=w52) -> (-x=w38:i32)
            n209 = local write "Y-Achse pos/neg fahren"(w38) -> ()
            n210 = Or(x=w46, y=w45) -> (x .or. y?=w44:bool)
            n211 = Equal?(x=w38, y=w42) -> (x = y?=w39:bool)
            n212 = Equal?(x=w38, y=w41) -> (x = y?=w40:bool)
            n213 = case shown="True" w44 {
              frame #0 {
              }
              frame #1 {
                n214 = local write "Achse in \nBewegung"(TRUE ("Achse in Bewegung")) -> ()
                n215 = local write "Joystickauslese"(T1."X-Achse" ("Joystickauslese")) -> ()
              }
            }
            n216 = Or(x=w39, y=w40) -> (x .or. y?=w37:bool)
            n217 = case shown="True" w37 {
              frame #0 {
              }
              frame #1 {
                n218 = local write "Achse in \nBewegung"(TRUE ("Achse in Bewegung")) -> ()
                n219 = local write "Joystickauslese"(T1."Y-Achse" ("Joystickauslese")) -> ()
              }
            }
          }
          frame #1 {
            n220 = control-ref of="Schrittweite [µm]"() -> (w68:refnum<vi>)
            n221 = property class="Ring (strikt)"(reference=w68) -> ("RingText.Text"=w69:string)  [unwired: 1 in, 2 out]
            n222 = local read "Joystickauslese"() -> (w70:T1)
            n223 = Fract/Exp String To Number(string=w69) -> (number=w67:dbl)  [unwired: 3 in, 1 out]
            n224 = case shown="\"Schrittweite verringern\"" w70 {
              tunnel: w67 -> [_ w73 w84 w89 w96 _ _]
              frame #0 {
              }
              frame #1 {
                n225 = local read "X-Achse pos/neg fahren"() -> (w76:i32)
                n226 = Multiply(x=w73, y=w76) -> (x*y=w75:dbl)
                n227 = local read "x-Achse"() -> (w74:i32)
                n228 = call "stage_move_axis_relative.vi"("Achse"=w74, "Schrittweite [µm]"=w75) -> ("error out"=w78:errorcluster, "Fertig?"=w77:bool, "xyz-Position OUT [mm]"=w71:dbl[])  [unwired: 1 in]
                n229 = local write "error out"(w78) -> ()
                n230 = local write "Aktuelle xyz-Position [mm]"(w71) -> ()
                n231 = local write "Ziel xyz-Position [mm]"(w71) -> ()
                n232 = Not(x=w77) -> (.not. x?=w72:bool)
                n233 = local write "Achse in \nBewegung"(w72) -> ()
              }
              frame #2 {
                n234 = local read "Y-Achse pos/neg fahren"() -> (w83:i32)
                n235 = Multiply(x=w84, y=w83) -> (x*y=w82:dbl)
                n236 = local read "y-Achse"() -> (w81:i32)
                n237 = call "stage_move_axis_relative.vi"("Achse"=w81, "Schrittweite [µm]"=w82) -> ("error out"=w86:errorcluster, "Fertig?"=w85:bool, "xyz-Position OUT [mm]"=w79:dbl[])  [unwired: 1 in]
                n238 = local write "error out"(w86) -> ()
                n239 = local write "Aktuelle xyz-Position [mm]"(w79) -> ()
                n240 = local write "Ziel xyz-Position [mm]"(w79) -> ()
                n241 = Not(x=w85) -> (.not. x?=w80:bool)
                n242 = local write "Achse in \nBewegung"(w80) -> ()
              }
              frame #3 {
                n243 = local read "z-Achse"() -> (w90:i32)
                n244 = call "stage_move_axis_relative.vi"("Achse"=w90, "Schrittweite [µm]"=w89) -> ("error out"=w92:errorcluster, "Fertig?"=w91:bool, "xyz-Position OUT [mm]"=w87:dbl[])  [unwired: 1 in]
                n245 = local write "error out"(w92) -> ()
                n246 = local write "Aktuelle xyz-Position [mm]"(w87) -> ()
                n247 = local write "Ziel xyz-Position [mm]"(w87) -> ()
                n248 = Not(x=w91) -> (.not. x?=w88:bool)
                n249 = local write "Achse in \nBewegung"(w88) -> ()
              }
              frame #4 {
                n250 = Negate(x=w96) -> (-x=w95:dbl)
                n251 = local read "z-Achse"() -> (w97:i32)
                n252 = call "stage_move_axis_relative.vi"("Achse"=w97, "Schrittweite [µm]"=w95) -> ("error out"=w99:errorcluster, "Fertig?"=w98:bool, "xyz-Position OUT [mm]"=w93:dbl[])  [unwired: 1 in]
                n253 = local write "error out"(w99) -> ()
                n254 = local write "Aktuelle xyz-Position [mm]"(w93) -> ()
                n255 = Not(x=w98) -> (.not. x?=w94:bool)
                n256 = local write "Achse in \nBewegung"(w94) -> ()
                n257 = local write "Ziel xyz-Position [mm]"(w93) -> ()
              }
              frame #5 {
                n258 = local read "Schrittweite [µm]"() -> (w100:u16)
                n259 = Decrement(x=w100) -> (x-1=w101:u16)
                n260 = local write "Schrittweite [µm]"(w101) -> ()
              }
              frame #6 {
                n261 = local read "Schrittweite [µm]"() -> (w102:u16)
                n262 = Increment(x=w102) -> (x+1=w103:u16)
                n263 = local write "Schrittweite [µm]"(w103) -> ()
              }
            }
          }
          frame #2 {
            n264 = local write "Joystickauslese"(T1."Nichts tun" ("Joystickauslese")) -> ()
          }
        }
        n265 = Wait (ms) "Wartezeit erhöht Programmstabilität"(milliseconds to wait=u32 200 ("Zu wartende ms")) -> ()  [unwired: 1 out]
        n266 = local read "Bühnen schließen"() -> (w36:bool)
      }
    }
    frame #2 {
      n267 = flat-sequence {
        frame #0 {
          n268 = local read "Joystick ID"() -> (w272:refnum<k1>)
          n269 = call-poly <vilib>:"Close Input Device.vi"("device ID"=w272) -> ("error out"=w273:errorcluster)  [unwired: 9 in]
          n270 = local write "error out"(w273) -> ()
        }
        frame #1 {
          # "Verbindung zu Bühnen schließen"
          n271 = local read "x-Achse"() -> (w276:i32)
          n272 = call "Close connection if open.vi"("System no."=w276, "Close DaisyChain"=TRUE) -> ("error out"=w280:errorcluster)  [unwired: 16 in, 1 out]
          n273 = local read "y-Achse"() -> (w275:i32)
          n274 = call "Close connection if open.vi"("System no."=w275, "Close DaisyChain"=TRUE, "error in"=w280) -> ("error out"=w281:errorcluster)  [unwired: 15 in, 1 out]
          n275 = local read "z-Achse"() -> (w274:i32)
          n276 = call "Close connection if open.vi"("System no."=w274, "Close DaisyChain"=TRUE, "error in"=w281) -> ("error out"=w278:errorcluster)  [unwired: 15 in, 1 out]
          n277 = local write "error out"(w278) -> ()
          n278 = Unbundle By Name(w278) -> ("status"=w277:bool)
          n279 = local write "Bühnen\ninitialisiert"(w277) -> ()
          n280 = global write "global_stage_initialised.vi" "Bühne initialisiert"(w277) -> ()
        }
      }
    }
  }
  n281 = Not(x=w2) -> (.not. x?=w1:bool)
  n282 = property on="Bühnen schließen" class="Boolesch (strikt)"("Value"=w1) -> ()  [unwired: 2 in, 2 out]
